vi "sub_vi_arduino_first_communication.vi"(8 "error in (no error)":errorcluster, 9 "write buffer":string, 10 "Reads number":i32, 11 "VISA resource name in":refnum<visa-resource-name>) -> (0 "error out":errorcluster, 1 "Reads array":dbl[](array[numeric]), 2 "Received data":string, 3 "VISA resource name out":refnum<visa-resource-name>)   [LabVIEW 2019]
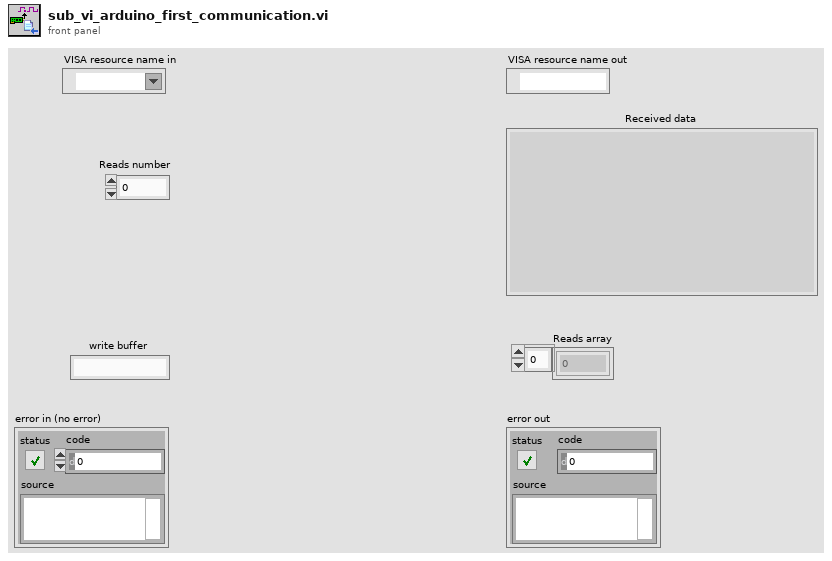
[diagram p1: front panel]
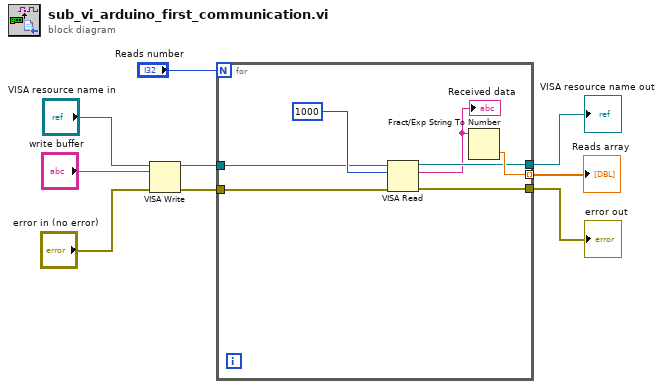
[diagram p0: block diagram]
diagram:
  n1 = VISA Write(VISA resource name="VISA resource name in", write buffer="write buffer", error in (no error)="error in (no error)") -> (VISA resource name out=w8:refnum<visa-resource-name>, error out=w9:errorcluster)  [unwired: 1 out]
  n2 = for {
    N: "Reads number" -> [_]
    tunnel: [w15] -> w3 mode=indexing
    tunnel: [w14] -> w1
    tunnel: [w16] -> w2
    tunnel: w9 -> [w11]
    tunnel: w8 -> [w10]
    n3 = VISA Read(VISA resource name=w10, byte count=u32 1000, error in (no error)=w11) -> (VISA resource name out=w14:refnum<visa-resource-name>, read buffer=w13:string, error out=w16:errorcluster)  [unwired: 1 out]
    "Received data" <- w13
    n4 = Fract/Exp String To Number(string=w13) -> (number=w15:dbl)  [unwired: 3 in, 1 out]
  }
  "Reads array" <- w3
  "error out" <- w2
  "VISA resource name out" <- w1
